vi "Actor Core.vi"(8 "error in":errorcluster, 11 "Unit_Test_Scope in":refnum<class "Unit_Test_Scope.lvclass">) -> (0 "error out":errorcluster, 3 "Actor out":refnum<class "Actor.lvclass">)   [LabVIEW 2020, in "Unit_Test_Scope.lvlib" / "Unit_Test_Scope.lvclass"]
doc: "(<B>Filename</B>: Actor Framework.lvlib:Actor.lvclass:Actor Core.vi)\n\nReceives messages to the actor, reacts to them, and initiates any error handling that may shut the actor down.\n\nDescendant classes may override this VI to append parallel tasks for the actor to complete while it handles messages. Overrides use the Call Parent Class Method node."
uses:
  Unit_Test_Scope.lvclass
  C:/Program Files/National Instruments/LabVIEW 2020/vi.lib/ActorFramework/Actor/Actor.lvclass
  <vilib>/ActorFramework/Actor/Actor.lvclass
  Actor_Scope/Actor_Scope/Actor_Scope.lvclass
  Unit_Test_Scope.lvclass/Unit_Test_Scope.ctl
  <vilib>/ActorFramework/Actor/Actor.lvclass/Actor.ctl
  <vilib>/ActorFramework/Message Enqueuer/Message Enqueuer.lvclass/Message Enqueuer.ctl
  <vilib>/ActorFramework/Stop Msg/Stop Msg.lvclass/Stop Msg.ctl
  Actor_Scope/Actor_Scope/Scope_Action.ctl
  Actor_Scope/Actor_Scope Messages/Do Scope Action Msg/Do Scope Action Msg.lvclass/Do Scope Action Msg.ctl
  <vilib>/ActorFramework/Message Enqueuer/Init from Existing Queue.vi
  <vilib>/ActorFramework/Stop Msg/Send Emergency Stop.vi
  <vilib>/ActorFramework/Stop Msg/Send Normal Stop.vi
  <vilib>/ActorFramework/Message Enqueuer/Enqueue.vi
  <vilib>/ActorFramework/Message Enqueuer/Enqueue Critical.vi
  <vilib>/ActorFramework/Stop Msg/Stop Msg.lvclass
  C:/Program Files/National Instruments/LabVIEW 2020/vi.lib/ActorFramework/Message/Message.lvclass
  Actor_Scope/Actor_Scope Messages/Do Scope Action Msg/Do Scope Action Msg.lvclass
  <vilib>/ActorFramework/Message Priority Queue/Priority Enqueue.vi
  <vilib>/ActorFramework/Message Enqueuer/Message Enqueuer.lvclass
panel:
  out "Resistance":dbl[](graph)
  out "Current Waveform":dbl[](graph)
  out "Voltage Wfm":dbl[](graph)
  in  "Time Out (ms)":i32=5000
  in  "Init Wfm Acq":bool
  out "log":string[](array[string])
  # "Scope Unit Test Front Panel"
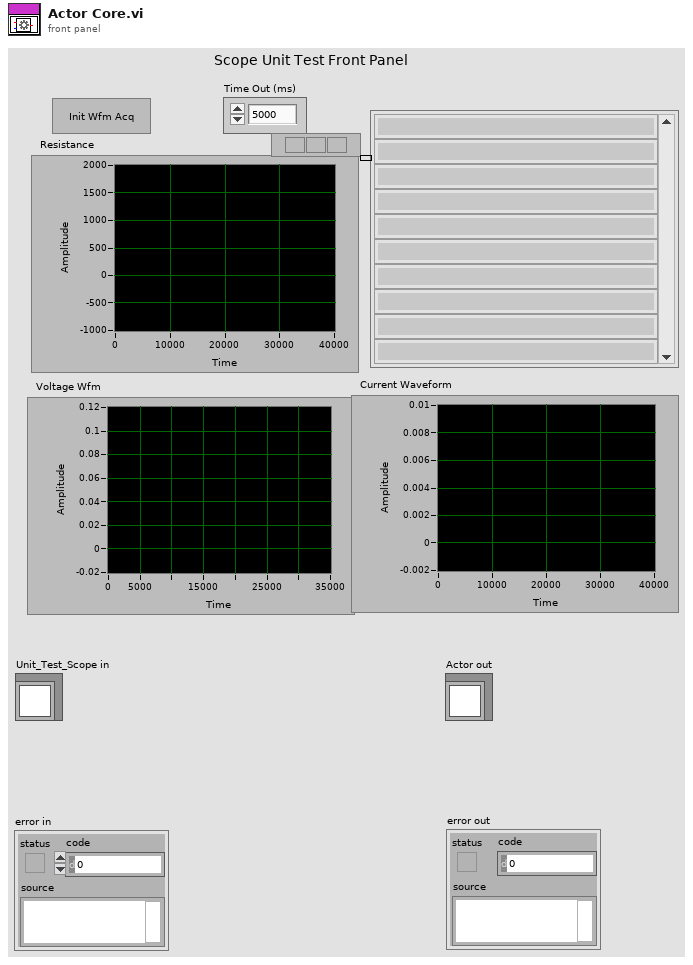
[diagram p1: front panel]
types:
  T1 = enum32{"Invalid", "Standard", "Closed", "Hidden", "Minimized", "Maximized"}
  T2 = typedef "Actor_Scope.lvlib/Actor_Scope.lvclass/Scope_Action.ctl" = enum16{"Config Trigger", "Init Wfm Acq", "Read Wfm"}
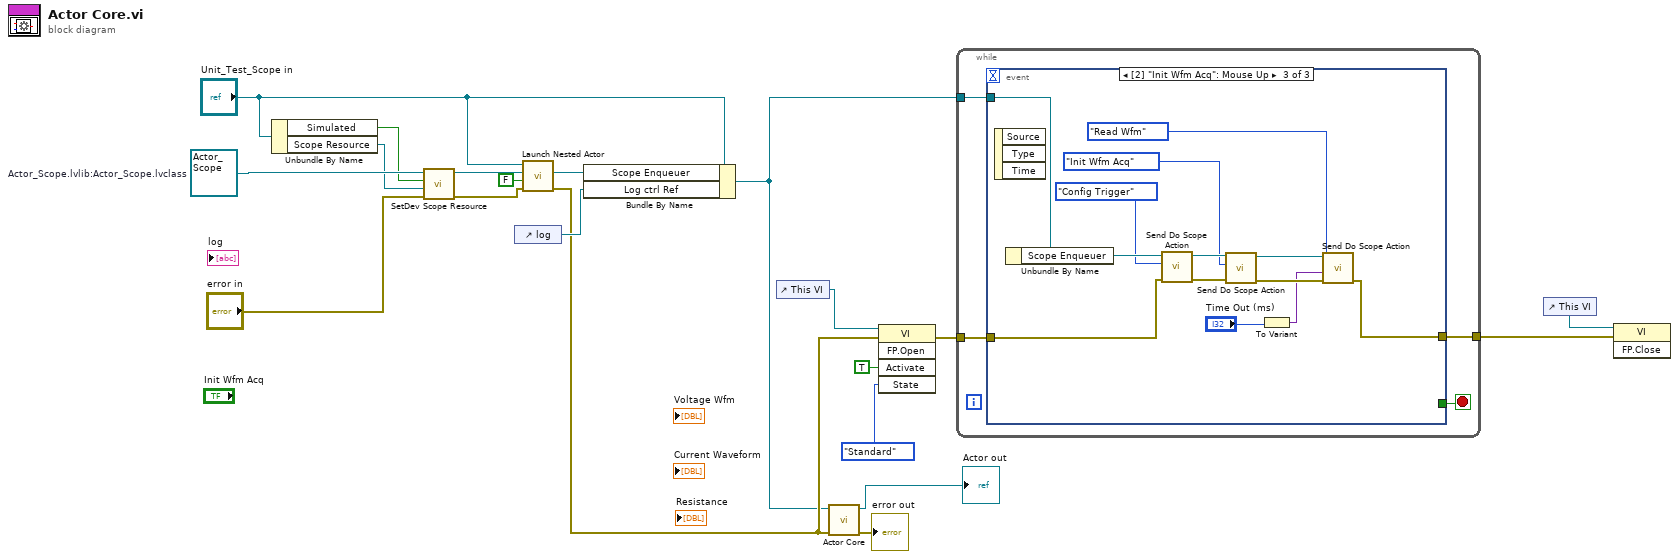
[diagram p0: block diagram]
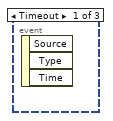
[diagram p2: hidden frame]
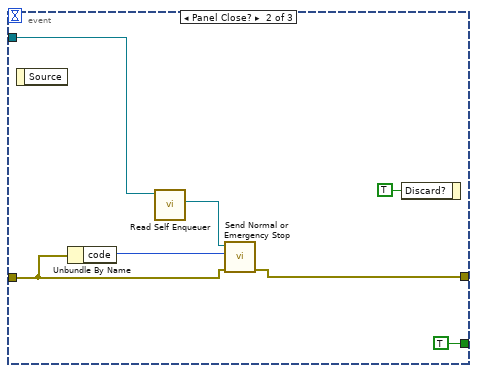
[diagram p3: hidden frame]
diagram:
  w18 = refnum<class "Actor_Scope.lvclass"> refnum  # Actor_Scope.lvlib:Actor_Scope.lvclass
  n1 = Unbundle By Name("Unit_Test_Scope in") -> ("Simulated"=w16:bool, "Scope Resource"=w17:refnum<visa-resource-name>)
  n2 = call-dynamic "SetDev Scope Resource.vi"("error in (no error)"="error in", "Scope VISA Addr"=w17, "Simulated"=w16, "Actor_Scope in"=w18) -> ("error out"=w12:errorcluster, "Actor_Scope out"=w14:refnum<class "Actor_Scope.lvclass">)  [unwired: 6 in]
  n3 = control-ref of="log"() -> (w10:refnum<vi>)
  n4 = call <vilib>:"Launch Nested Actor.vi"("error in (no error)"=w12, "Auto-stop? (T)"=FALSE, "Nested Actor"=w14, "Caller Actor in"="Unit_Test_Scope in") -> ("error out"=w5:errorcluster, "Nested Actor's Enqueuer"=w11:refnum<class "Message Enqueuer.lvclass">)  [unwired: 5 in, 1 out]
  n5 = Bundle By Name(cluster="Unit_Test_Scope in", "Scope Enqueuer"=w11, "Log ctrl Ref"=w10) -> (w4:refnum<class "Unit_Test_Scope.lvclass">)
  n6 = control-ref of="This VI"() -> (w8:refnum<vi>)
  n7 = call-parent "Actor Core.vi"("error in"=w5, "Actor in"=w4) -> ("error out"=→"error out":errorcluster, "Actor out"=→"Actor out":refnum<class "Actor.lvclass">)  [unwired: 8 in]
  n8 = invoke class="VI" method="FP.Open"(reference=w8, error in=w5, "Activate"=TRUE ("Activate?"), "State"=T1."Standard") -> (error out=w3:errorcluster)  [unwired: 1 in, 4 out]
  n9 = while {
    tunnel: w4 -> [w23]
    tunnel: w3 -> [w24]
    tunnel: [w22] -> w1
    stop <- w21 stop-if-true
    n10 = event shown="[2] \"Init Wfm Acq\": Mouse Up" {
      selector: _ -> [_ _ _]
      dyn-events: _ -> [_ _ _]
      timeout: _ -> [_ _ _]
      tunnel: w24 -> [_ w27 w41]
      tunnel: w23 -> [_ w30 w44]
      tunnel: [_ w26 w32] -> w22
      tunnel: [_ TRUE _] -> w21
      event Timeout {
        n11 = event-data() -> ()  [unwired: 1 in, 3 out]
      }
      event Panel Close? {
        n12 = event-data() -> ()  [unwired: 1 in, 1 out]
        n13 = Unbundle By Name(w27) -> ("code"=w29:i32)
        n14 = call <vilib>:"Read Self Enqueuer.vi"("Actor"=w30) -> ("Self Enqueuer"=w28:refnum<class "Message Enqueuer.lvclass">)  [unwired: 10 in]
        n15 = call <vilib>:"Send Normal or Emergency Stop.vi"("error in (no error)"=w27, "final error code"=w29, "Message Enqueuer"=w28) -> ("error out"=w26:errorcluster)  [unwired: 8 in]
        n16 = event-data("Discard?"=TRUE) -> ()  [unwired: 1 in, 1 out]
      }
      event "Init Wfm Acq": Mouse Up {
        n17 = event-data() -> ()  [unwired: 1 in, 3 out]
        n18 = Unbundle By Name(w44) -> ("Scope Enqueuer"=w43:refnum<class "Message Enqueuer.lvclass">)
        n19 = call "Send Do Scope Action.vi"("error in (no error)"=w41, "Scope Action"=Scope_Action."Config Trigger", "Message Enqueuer"=w43) -> ("error out"=w39:errorcluster, "Message Enqueuer out"=w40:refnum<class "Message Enqueuer.lvclass">)  [unwired: 7 in]
        n20 = call "Send Do Scope Action.vi"("error in (no error)"=w39, "Scope Action"=Scope_Action."Init Wfm Acq", "Message Enqueuer"=w40) -> ("error out"=w36:errorcluster, "Message Enqueuer out"=w37:refnum<class "Message Enqueuer.lvclass">)  [unwired: 7 in]
        n21 = To Variant(anything="Time Out (ms)") -> (Variant=w33:variant)
        n22 = call "Send Do Scope Action.vi"("error in (no error)"=w36, "Action Data In"=w33, "Scope Action"=Scope_Action."Read Wfm", "Message Enqueuer"=w37) -> ("error out"=w32:errorcluster)  [unwired: 6 in, 1 out]
      }
    }
  }
  n23 = control-ref of="This VI"() -> (w2:refnum<vi>)
  n24 = invoke class="VI" method="FP.Close"(reference=w2, error in=w1) -> ()  [unwired: 1 in, 3 out]
